vi "UpdateSelectStatus.vi"(7 "Available Points":refnum<vi>, 8 "error in (no error)":errorcluster, 10 "Available Points Idx":T1) -> (0 "error out":errorcluster)   [LabVIEW 2019]
uses:
  <vilib>/Utility/miscctls.llb/LVRowAndColumnTypeDef.ctl
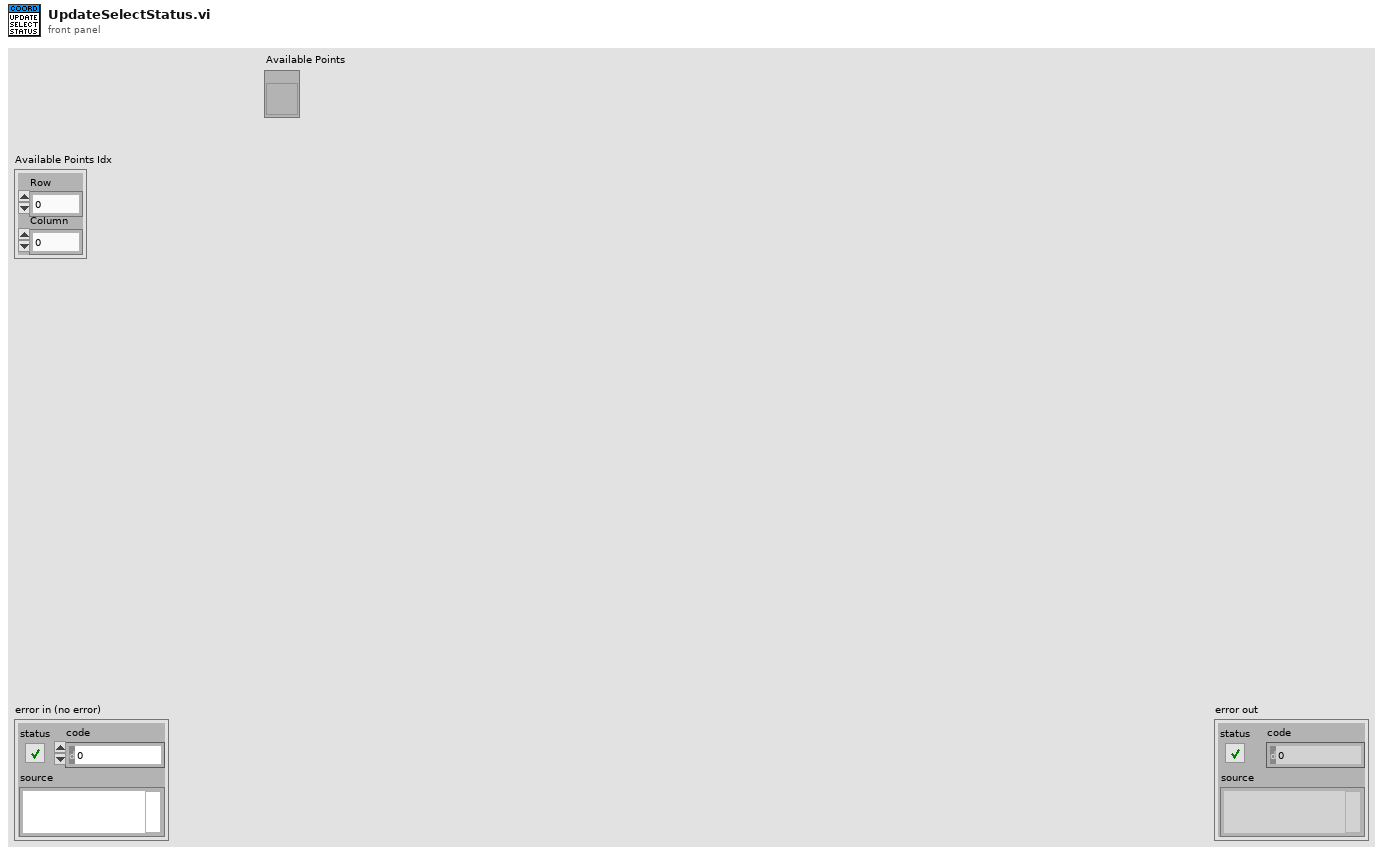
[diagram p1: front panel]
types:
  T1 = typedef "LVRowAndColumnTypeDef.ctl" = cluster{"Row":i32, "Column":i32}
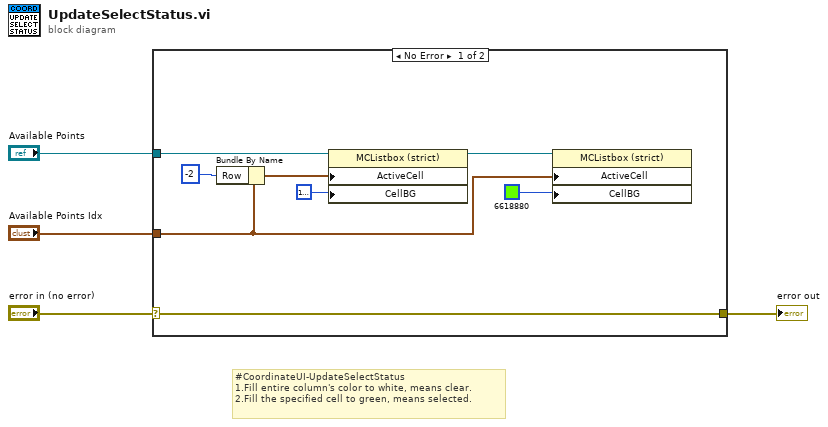
[diagram p0: block diagram]
diagram:
  # "#CoordinateUI-UpdateSelectStatus\n1.Fill entire column's color to white, means clear.\n2.Fill the specified cell to green, means selected."
  n1 = case shown="No Error" "error in (no error)" {
    selector: "error in (no error)" -> [w5 w13]
    tunnel: "Available Points" -> [w12 _]
    tunnel: "Available Points Idx" -> [w8 _]
    tunnel: [w5 w13] -> w1
    frame No Error {
      n2 = Bundle By Name(cluster=w8, "Row"=-2) -> (w9:T1)
      n3 = property class="MCListbox (strict)"(reference=w12, "ActiveCell"=w9, "CellBG"=u32 16777225) -> (reference out=w11:refnum<vi>)  [unwired: 1 in, 1 out]
      n4 = property class="MCListbox (strict)"(reference=w11, "ActiveCell"=w8, "CellBG"=u32 6618880) -> ()  [unwired: 1 in, 2 out]
    }
    frame Error {
    }
  }
  "error out" <- w1
